vi "Init Panel.vi"(8 "error in (no error)":errorcluster, 11 "vi reference":refnum<vi>) -> (0 "error out":errorcluster, 3 "vi reference (out)":refnum<vi>)   [LabVIEW 2017, in "WebServiceImporter.lvlib" / "Main Panel.lvlib"]
uses:
  <vilib>/Platform/WebService/Main Panel/Main Panel.lvlib
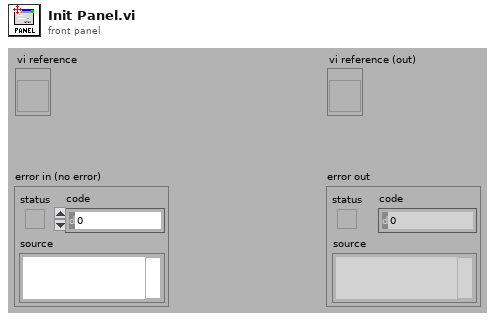
[diagram p1: front panel]
types:
  T1 = typedef "LVRectTypeDef.ctl" = cluster{"Left":i16, "Top":i16, "Right":i16, "Bottom":i16}
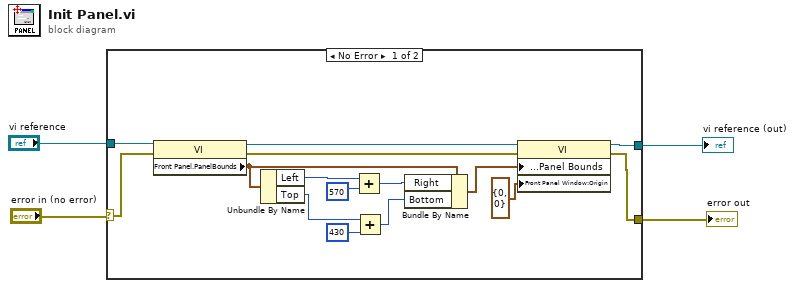
[diagram p0: block diagram]
diagram:
  n1 = case shown="No Error" "error in (no error)" {
    selector: "error in (no error)" -> [w18 w21]
    tunnel: "vi reference" -> [w19 w20]
    tunnel: [w8 w20] -> w2
    tunnel: [w7 w21] -> w1
    frame No Error {
      n2 = property class="VI"(reference=w19, error in=w18) -> (reference out=w10:refnum<vi>, error out=w9:errorcluster, "Front Panel.PanelBounds"=w17:T1)
      n3 = Unbundle By Name(w17) -> ("Left"=w16:i16, "Top"=w13:i16)
      n4 = Add(x=w16, y=i16 570) -> (x+y=w14:i16)
      n5 = Add(x=w13, y=i16 430) -> (x+y=w11:i16)
      n6 = Bundle By Name(cluster=w17, "Right"=w14, "Bottom"=w11) -> (w6:T1)
      n7 = property class="VI"(reference=w10, error in=w9, "Front Panel Window:Panel Bounds"=w6, "Front Panel Window:Origin"=cluster{"Horizontal":i16, "Vertical":i16} {"Horizontal"=0, "Vertical"=0}) -> (reference out=w8:refnum<vi>, error out=w7:errorcluster)
    }
    frame Error {
    }
  }
  "error out" <- w1
  "vi reference (out)" <- w2
